vi "combined arm safety.vi"(7 "Input":dbl) -> (8 "Safe Output":dbl, 13 "Safety Data":T1)   [LabVIEW 2013]
uses:
  typedefs/dashboard safety status data.ctl
  typedefs/DevRef Type.ctl
  typedefs/fg_typedef.ctl
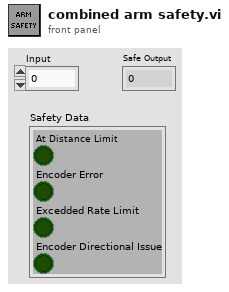
[diagram p1: front panel]
types:
  T1 = typedef "dashboard safety status data.ctl" = cluster{"At Distance Limit":bool, "Encoder Error":bool, "Excedded Rate Limit":bool, "Encoder Directional Issue":bool}
  T2 = typedef "fg_typedef.ctl" = enum16{"Get", "Set"}
  T3 = typedef "DevRef Type.ctl" = enum16{"Shooter Solenoid", "Latch Solenoid", "Right Up Sensor", "Right Down Sensor", "Hold Sensor", "2 Ball Switch", "Arm Encoder"}
  T4 = typedef "WPI_EncoderDevRef.ctl" = cluster{"DevStatus":errorcluster, "EncoderIndex":T5, "CounterIndex":T6, "DistancePerCount":dbl, "Decoding Type":T7}
  T5 = typedef "FPGA_EncoderIdx.ctl" = enum8{"Enc 0", "Enc 1", "Enc 2", "Enc 3", "Invalid"}
  T6 = typedef "FPGA_CounterCtrSystemIndex.ctl" = enum8{"Ctr 0", "Ctr 1", "Ctr 2", "Ctr 3", "Ctr 4", "Ctr 5", "Ctr 6", "Ctr 7", "Invalid"}
  T7 = typedef "WPI_EncoderType.ctl" = enum16{"1x", "2x", "4x"}
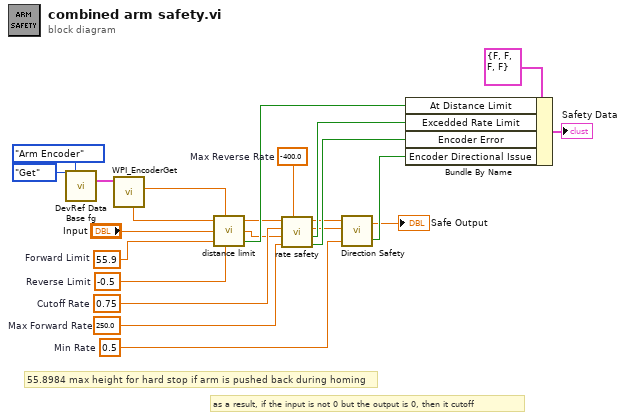
[diagram p0: block diagram]
diagram:
  w7 = 250.0  # Max Forward Rate
  w8 = -400.0  # Max Reverse Rate
  w4 = 0.5  # Min Rate
  w9 = 0.75  # Cutoff Rate
  w11 = -0.5  # Reverse Limit
  w12 = 55.9  # Forward Limit
  # "55.8984 max height for hard stop if arm is pushed back during homing"
  # "as a result, if the input is not 0 but the output is 0, then it cutoff"
  n1 = call "DevRef Data Base fg.vi"("Menu"=fg_typedef."Get", "DevRef to Get"=DevRef_Type."Arm Encoder") -> ("Selected Encoder"=w16:T4)  [unwired: 23 in, 2 out]
  n2 = call <vilib>:"WPI_EncoderGet.vi"("EncoderDevRef"=w16) -> ("Distance"=w14:dbl, "Rate"=w15:dbl)  [unwired: 5 in, 4 out]
  n3 = call "distance limit.vi"("Encoder Rate"=w15, "Encoder Distance"=w14, "Desired Rate"="Input", "Forward Limit"=w12, "Reverse Limit"=w11) -> ("Encoder Rate Out"=w10:dbl, "Output Rate"=w2:dbl, "At Distance Limit"=w22:bool)
  n4 = call "rate safety.vi"("Max Reverse Rate"=w8, "Max Forward Rate"=w7, "Desired Rate"=w2, "Cutoff Rate"=w9, "Encoder Rate"=w10) -> ("Encoder Error"=w20:bool, "Excedded Rate Limit"=w21:bool, "Output Rate"=w5:dbl, "Encoder Rate Out"=w6:dbl)
  n5 = call "Direction Safety.vi"("Min Rate"=w4, "Desired Rate"=w5, "Encoder Rate"=w6) -> ("Encoder Directional Issue"=w23:bool, "Super Safe Rate"=→"Safe Output":dbl)
  n6 = Bundle By Name(cluster=T1 {"At Distance Limit"=FALSE, "Encoder Error"=FALSE, "Excedded Rate Limit"=FALSE, "Encoder Directional Issue"=FALSE} ("Input"), "At Distance Limit"=w22, "Excedded Rate Limit"=w21, "Encoder Error"=w20, "Encoder Directional Issue"=w23) -> (→"Safety Data":T1)
